vi "Read.vi"(5 "CS Channel":u8, 7 "SPI Channel (0)":u8, 8 "Error In":errorcluster, 10 "Supply Voltage":dbl, 11 "LINX Resource":T1) -> (0 "Error Out":errorcluster, 2 "Voltage (V)":dbl, 3 "LINX Resource":T1)   [LabVIEW 2020, in "LMH-LINX.lvlib" / "PmodMIC3.lvlib"]
doc: "Read the voltage from the PmodMIC3."
uses:
  PmodMIC3.lvlib
  Private/Type Defs/LINX Ref.ctl
  Private/Type Defs/Platform.ctl
  Private/Type Defs/Interface.ctl
  Private/Device/Type Defs/LINX Device Config.ctl
  Private/Device/Type Defs/TCP Config.ctl
  Private/Device/Type Defs/Channels.ctl
  Peripherals/SPI/SPI CS Config.ctl
  Private/Type Defs/Peripherals/SPI/SPI CS Logic Level.ctl
  Peripherals/SPI/SPI Write Read 1 Frame.vi
  Peripherals/SPI/SPI Write Read N Frames.vi
  Utilities/Check Channel.vi
  Private/Utilties/Generate Error.vi
  LMH-LINX.lvlib
  Private/Device/Device.lvlib
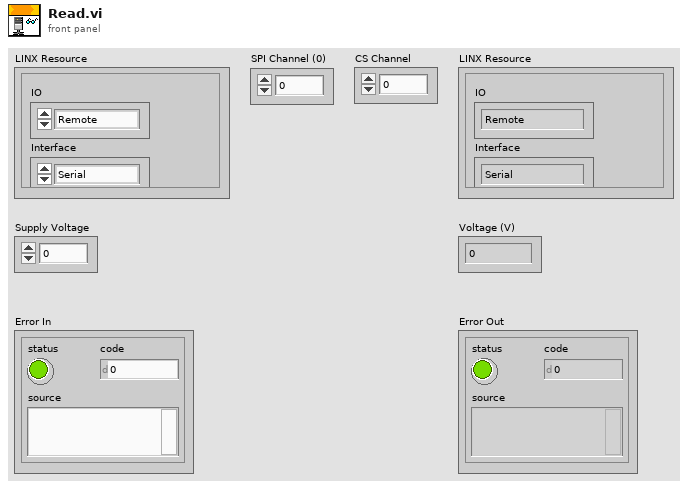
[diagram p1: front panel]
types:
  T1 = typedef "LMH-LINX.lvlib/LINX Ref.ctl" = cluster{"IO":T2, "Interface":T3, "LINX Device Config":T4}
  T2 = typedef "LMH-LINX.lvlib/Platform.ctl" = enum16{"Remote", "Local"}
  T3 = typedef "LMH-LINX.lvlib/Interface.ctl" = enum16{"Serial", "TCP"}
  T4 = typedef "Device.lvlib/LINX Device Config.ctl" = cluster{"Interface":T3, "COM Port":refnum<visa-resource-name>, "TCP Configuration":T5, "Device Family":u8, "Device ID":u8, "Device Name":string, "TCP Ref":refnum<k5>, "Channels":T6}
  T5 = typedef "Device.lvlib/TCP Config.ctl" = cluster{"IP Address":string, "Port":u16}
  T6 = typedef "LMH-LINX.lvlib/Channels.ctl" = cluster{"DI":u8[], "DO":u8[], "AI":u8[], "AO":u8[], "PWM":u8[], "QE":u8[], "UART":u8[], "I2C 2":u8[], "SPI":u8[], "CAN":u8[], "Servo":u8[], "AI Ref (V)":dbl, "AI Resolution (Bits)":u8, "AO Ref (V)":dbl, "AO Resolution (Bits)":u8}
  T7 = typedef "LMH-LINX.lvlib/SPI CS Config.ctl" = cluster{"CS Channel":u8, "CS Logic Level":T8}
  T8 = typedef "LMH-LINX.lvlib/SPI CS Logic Level.ctl" = enum8{"Active Low", "Active High"}
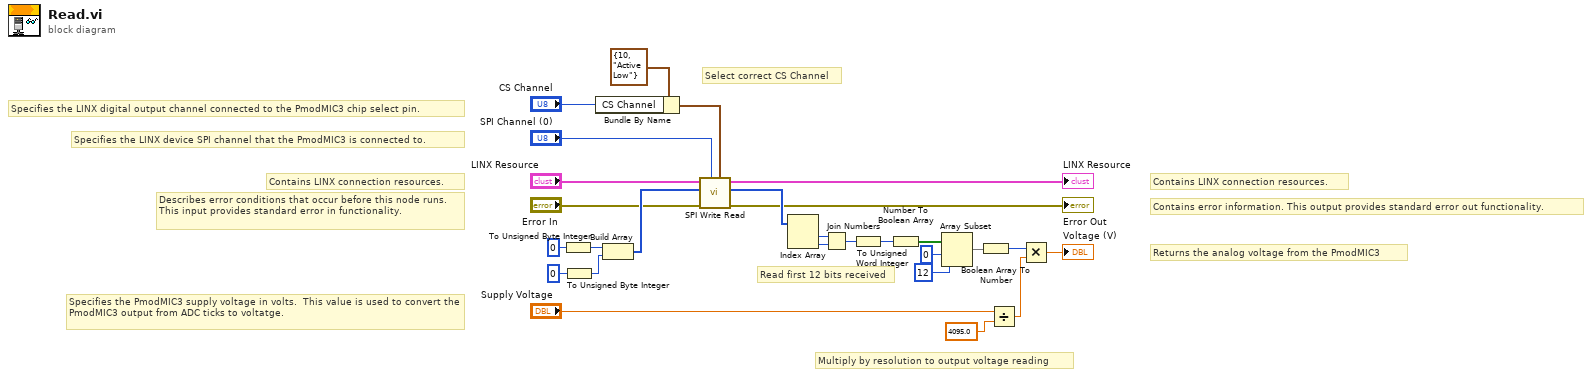
[diagram p0: block diagram]
diagram:
  # "Specifies the LINX device SPI channel that the PmodMIC3 is connected to."
  # "Specifies the LINX digital output channel connected to the PmodMIC3 chip select pin."
  # "Specifies the PmodMIC3 supply voltage in volts.  This value is used to convert the PmodMIC3 output from ADC ticks to voltatge."
  # "Returns the analog voltage from the PmodMIC3"
  # "Contains LINX connection resources."
  # "Contains error information. This output provides standard error out functionality."
  # "Contains LINX connection resources."
  # "Describes error conditions that occur before this node runs. This input provides standard error in functionality."
  # "Multiply by resolution to output voltage reading"
  # "Read first 12 bits received"
  # "Select correct CS Channel"
  n1 = To Unsigned Byte Integer(number=0) -> (unsigned 8bit integer=w10:u8)
  n2 = To Unsigned Byte Integer(number=0) -> (unsigned 8bit integer=w9:u8)
  n3 = Bundle By Name(cluster=T7 {"CS Channel"=10, "CS Logic Level"=enum."Active Low"} ("CS Configuration"), "CS Channel"="CS Channel") -> (w1:T7)
  n4 = Build Array(w10, w9) -> (w11:u8[])
  n5 = call-poly "SPI Write Read.vi"("CS Configuration"=w1, "SPI Channel (0)"="SPI Channel (0)", "Error In"="Error In", "Data"=w11, "LINX Resource"="LINX Resource") -> ("Error Out"=→"Error Out":errorcluster, "Read Data"=w20:u8[], "LINX Resource"=→"LINX Resource":T1)  [unwired: 3 in, 1 out]
  n6 = Index Array(array=w20) -> (element #1=w13:u8, element #2=w14:u8)  [unwired: 2 in]
  n7 = Join Numbers(hi=w13, lo=w14) -> ((hi.lo)=w12:u16)
  n8 = To Unsigned Word Integer(number=w12) -> (unsigned 16bit integer=w15:u16)
  n9 = Number To Boolean Array(number=w15) -> (Boolean array=w16:bool[])
  n10 = Array Subset(array=w16, index=0, length=12) -> (w19:bool[])
  n11 = Boolean Array To Number(Boolean array=w19) -> (number=w21:u16)
  n12 = Divide(x="Supply Voltage", y=4095.0) -> (x/y=w24:dbl)
  n13 = Multiply(x=w21, y=w24) -> (x*y=→"Voltage (V)":dbl)
